vi "WPI_DMAAddChannelToStream_Timestamp.vi"(8 "error in (no error)":errorcluster, 11 "DMARef":T1) -> (0 "error out":errorcluster, 3 "DMARef":T1)   [LabVIEW 2017]
doc: "Adds a record of the FPGA clock to the DMA stream. Use this VI to learn when each sample was sent.\n\nThis software is licensed. Open the labview\\readme\\WPI Robotics Library Open Source License.txt file for more information."
uses:
  <vilib>/Rock Robotics/WPI/DMA/WPI_DMARef.ctl
  <vilib>/Rock Robotics/WPI/DMA/WPI_DMAChannelTypeEnum.ctl
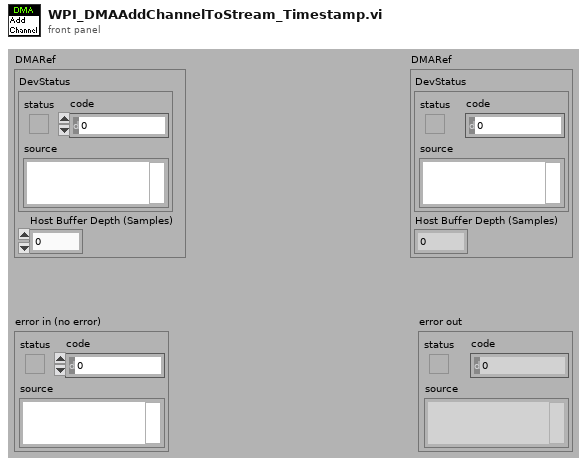
[diagram p1: front panel]
types:
  T1 = typedef "WPI_DMARef.ctl" = cluster{"DevStatus":errorcluster, "Host Buffer Depth (Samples)":u32}
  T2 = typedef "WPI_DMAChannelTypeEnum.ctl" = enum16{"AI (Raw)", "AI (Avg)", "Accumulator", "DI (Raw) Onboard", "DI (Filtered) Onboard", "DI (Raw) MXP", "DI (Filtered) MXP", "Analog Trigger", "Counter", "Counter (Timer)", "Encoder", "Encoder (Timer)", "Time Stamp"}
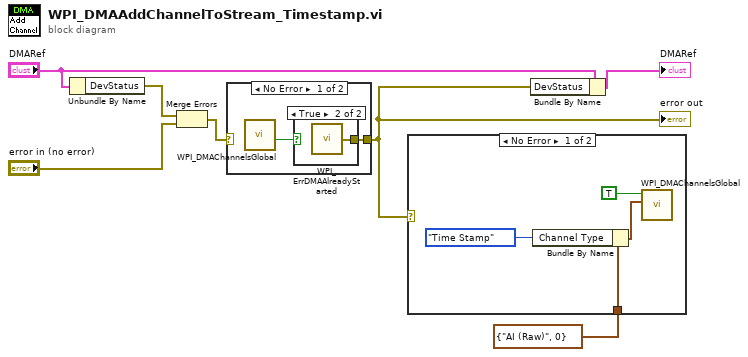
[diagram p0: block diagram]
diagram:
  n1 = Unbundle By Name("DMARef") -> ("DevStatus"=w2:errorcluster)
  n2 = Merge Errors(w2, "error in (no error)") -> (w1:errorcluster)
  n3 = case shown="No Error" w1 {
    selector: w1 -> [_ w11]
    tunnel: [w8 w11] -> w6
    frame No Error {
      n4 = call <vilib>:"WPI_DMAChannelsGlobal.vi"() -> ("Started"=w9:bool)  [unwired: 4 in, 7 out]
      n5 = case shown="True" w9 {
        tunnel: [_ w10] -> w8
        frame False {
        }
        frame True {
          n6 = call <vilib>:"WPI_ErrDMAAlreadyStarted.vi"() -> ("error out"=w10:errorcluster)
        }
      }
    }
    frame Error {
    }
  }
  "error out" <- w6
  n7 = case shown="No Error" w6 {
    tunnel: cluster{"Channel Type":T2, "Channel Number":u8} {"Channel Type"=enum."AI (Raw)", "Channel Number"=0} ("Channel") -> [w14 _]
    frame No Error {
      n8 = Bundle By Name(cluster=w14, "Channel Type"=WPI_DMAChannelTypeEnum."Time Stamp") -> (w13:cluster{"Channel Type":T2, "Channel Number":u8})
      n9 = call <vilib>:"WPI_DMAChannelsGlobal.vi"("Channel"=w13, "Add"=TRUE) -> ()  [unwired: 2 in, 8 out]
    }
    frame Error {
    }
  }
  n10 = Bundle By Name(cluster="DMARef", "DevStatus"=w6) -> (→"DMARef":T1)
